vi "字符键盘.vi"(10 "显示样式":u32, 11 "原值":string) -> (3 "x+y":string)   [LabVIEW 2016, in "斯坦道CODMn.lvlib"]
uses:
  <vilib>/event_ctls.llb/eventvkey.ctl
panel:
  in  "CapsLock":bool
  in  "M":bool
  in  "N":bool
  in  "B":bool
  in  "V":bool
  in  "C":bool
  in  "X":bool
  in  "Z":bool
  in  "L":bool
  in  "K":bool
  in  "J":bool
  in  "H":bool
  in  "G":bool
  in  "F":bool
  in  "D":bool
  in  "S":bool
  in  "A":bool
  in  "P":bool
  in  "O":bool
  in  "I":bool
  in  "U":bool
  in  "Y":bool
  in  "T":bool
  in  "R":bool
  in  "E":bool
  in  "W":bool
  in  "Q":bool
  in  "清除":bool
  in  "退格":bool
  in  "取消按钮":bool
  in  ".":bool
  out "字符串":string
  in  "0":bool
  in  "停止":bool
  in  "9":bool
  in  "8":bool
  in  "7":bool
  in  "6":bool
  in  "5":bool
  in  "4":bool
  in  "3":bool
  in  "2":bool
  in  "1":bool
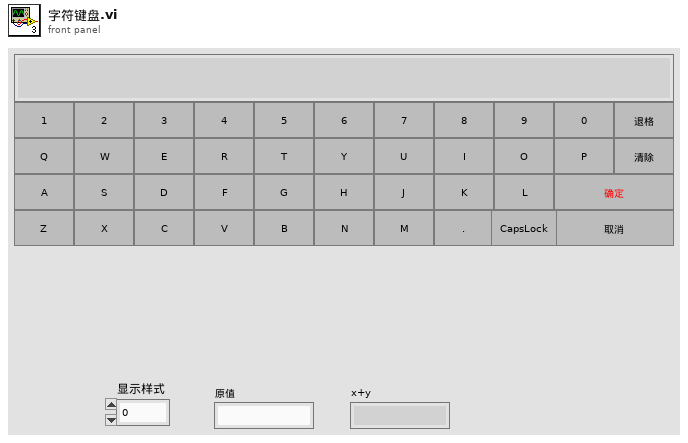
[diagram p1: front panel]
types:
  T1 = typedef "eventvkey.ctl" = enum16{"ASCII", "Enter", "Return", "Shift", "Ctrl", "Alt", "Cmd", "Opt", "Caps", "NumLock", "Clear", "Break", "Up", "Down", "Left", "Right", "Insert", "Delete", "Home", "End", "PageUp", "PageDown", "Escape", "Help", "Pause", "ScrollLock", "F1", "F2", "F3", "F4", "F5", "F6", "F7", "F8", "F9", "F10", "F11", "F12", "F13", "F14", "F15", "F16", "F17", "F18", "F19", "F20", "F21", "F22", "F23", "F24", "Play", "VolumeUp", "VolumeDown", "Mute", "Two Byte Char"}
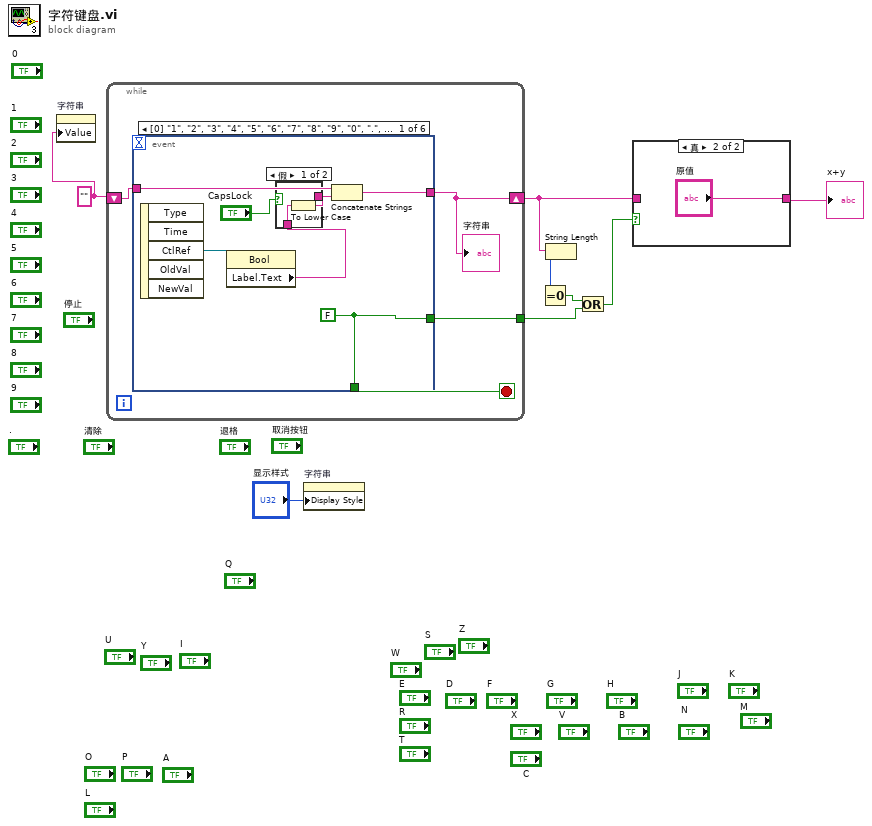
[diagram p0: block diagram]
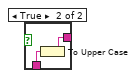
[diagram p3: hidden frame]
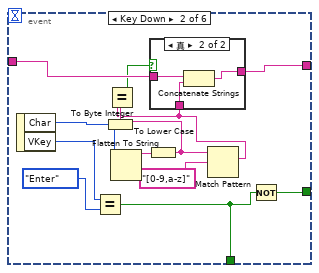
[diagram p4: hidden frame]
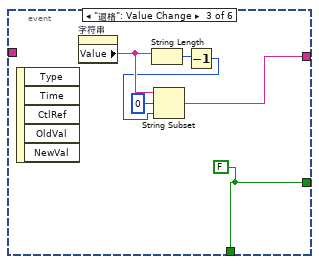
[diagram p6: hidden frame]
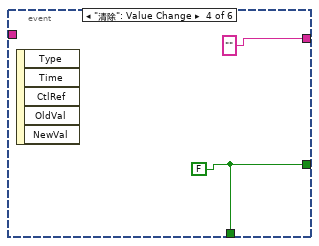
[diagram p7: hidden frame]
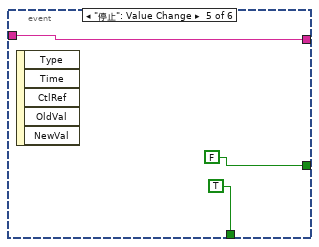
[diagram p8: hidden frame]
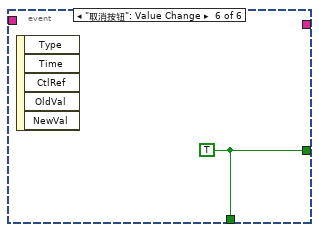
[diagram p9: hidden frame]
diagram:
  w8 = "" ("Label.Text")
  n1 = property on="字符串" class="Str"("Value"=w8) -> ()  [unwired: 2 in, 2 out]
  n2 = while {
    shift-right: [w11] -> w7
    shift-left: w8 -> [w10]
    tunnel: [w9] -> w2
    stop <- w12 stop-if-true
    n3 = event shown="[0] \"1\", \"2\", \"3\", \"4\", \"5\", \"6\", \"7\", \"8\", \"9\", \"0\", \".\", \"Q\", \"W\", \"E\", \"R\", \"T\", \"Y\", \"U\", \"I\", \"O\", \"P\", \"A\", \"S\", \"D\", \"F\", \"G\", \"H\", \"J\", \"K\", \"L\", \"Z\", \"X\", \"C\", \"V\", \"B\", \"N\", \"M\": 值改变" {
      selector: _ -> [_ _ _ _ _ _]
      dyn-events: _ -> [_ _ _ _ _ _]
      timeout: _ -> [_ _ _ _ _ _]
      tunnel: [w16 w25 w41 w47 TRUE w52] -> w12
      tunnel: [w18 w33 w42 "" ("Label.Text") w50 _] -> w11
      tunnel: w10 -> [w17 w32 _ _ w50 _]
      tunnel: [w16 w26 w41 w47 FALSE w52] -> w9
      event "1", "2", "3", "4", "5", "6", "7", "8", "9", "0", ".", "Q", "W", "E", "R", "T", "Y", "U", "I", "O", "P", "A", "S", "D", "F", "G", "H", "J", "K", "L", "Z", "X", "C", "V", "B", "N", "M": Value Change {
        w16 = FALSE
        n4 = event-data() -> ("CtlRef"=w19:refnum<vi>)  [unwired: 1 in, 4 out]
        n5 = property class="Bool"(reference=w19) -> ("Label.Text"=w14:string)  [unwired: 1 in, 2 out]
        n6 = case shown="假" "CapsLock" {
          tunnel: [w21 w22] -> w15
          tunnel: w14 -> [w20 w23]
          frame False {
            n7 = To Lower Case(string=w20) -> (all lower case string=w21:string)
          }
          frame True {
            n8 = To Upper Case(1:w23) -> (0:w22:string)
          }
        }
        n9 = Concatenate Strings(w17, w15) -> (w18:string)
      }
      event Key Down {
        n10 = event-data() -> ("Char"=w36:i16, "VKey"=w24:T1)  [unwired: 1 in]
        n11 = Equal?(x=w24, y=eventvkey."Enter" ("V键")) -> (x = y?=w25:bool)
        n12 = To Byte Integer(number=w36) -> (8bit integer=w35:i8)
        n13 = Flatten To String(anything=w35) -> (data string=w34:string)  [unwired: 3 in, 2 out]
        n14 = To Lower Case(string=w34) -> (all lower case string=w30:string)
        n15 = Match Pattern(string=w30, regular expression="[0-9,a-z]" ("正则表达式")) -> (match substring=w29:string)  [unwired: 1 in, 3 out]
        n16 = Equal?(x=w30, y=w29) -> (x = y?=w28:bool)
        n17 = case shown="真" w28 {
          tunnel: [w37 w40] -> w33
          tunnel: w32 -> [w37 w39]
          tunnel: w29 -> [_ w38]
          frame False {
          }
          frame True {
            n18 = Concatenate Strings(w39, w38) -> (w40:string)
          }
        }
        n19 = Not(x=w25) -> (.not. x?=w26:bool)
      }
      event "退格": Value Change {
        w41 = FALSE
        n20 = event-data() -> ()  [unwired: 1 in, 5 out]
        n21 = property on="字符串" class="Str"() -> ("Value"=w45:string)  [unwired: 2 in, 2 out]
        n22 = String Length(string=w45) -> (length=w46:i32)
        n23 = Decrement(x=w46) -> (x-1=w43:i32)
        n24 = String Subset(string=w45, offset (0)=0 ("偏移量(0)"), length (rest)=w43) -> (substring=w42:string)
      }
      event "清除": Value Change {
        w47 = FALSE
        n25 = event-data() -> ()  [unwired: 1 in, 5 out]
      }
      event "停止": Value Change {
        n26 = event-data() -> ()  [unwired: 1 in, 5 out]
      }
      event "取消按钮": Value Change {
        w52 = TRUE
        n27 = event-data() -> ()  [unwired: 1 in, 5 out]
      }
    }
    "字符串" <- w11
  }
  n28 = property on="字符串" class="Str"("Display Style"="显示样式") -> ()  [unwired: 2 in, 2 out]
  n29 = String Length(string=w7) -> (length=w6:i32)
  n30 = Equal To 0?(x=w6) -> (x = 0?=w5:bool)
  n31 = Or(x=w5, y=w2) -> (x .or. y?=w4:bool)
  n32 = case shown="真" w4 {
    tunnel: w7 -> [w53 _]
    tunnel: [w53 "原值"] -> w3
    frame False {
    }
    frame True {
    }
  }
  "x+y" <- w3
